vi "Resolve ByteCount Wait.vi"(8 "error in (no error)":errorcluster, 11 "Settings in":T1 {"Channel Refnum" format="%.0x"; "Linked Channels"."Channel Refnum" format="%.0x"}) -> (0 "error out":errorcluster, 1 "Byte Count":i32, 2 "Channel Path":string, 3 "Settings out":T1 {"Channel Refnum" format="%.0x"; "Linked Channels"."Channel Refnum" format="%.0x"})   [LabVIEW 2020, in "Instrument Addon Scripting API.lvlib"]
uses:
  Instrument Addon Scripting API.lvlib
  TypeDefs/ByteCount Response Settings.ctl
  TypeDefs/Linked Channel.ctl
  <vilib>/NI VeriStand/Custom Device API/Custom Device Item Ref.ctl
  NationalInstruments.VeriStand.SystemStorage
  Shared Directory/Instrument Addon Shared.lvlib
  <vilib>/NI VeriStand/Custom Device API/Custom Device API.lvlib
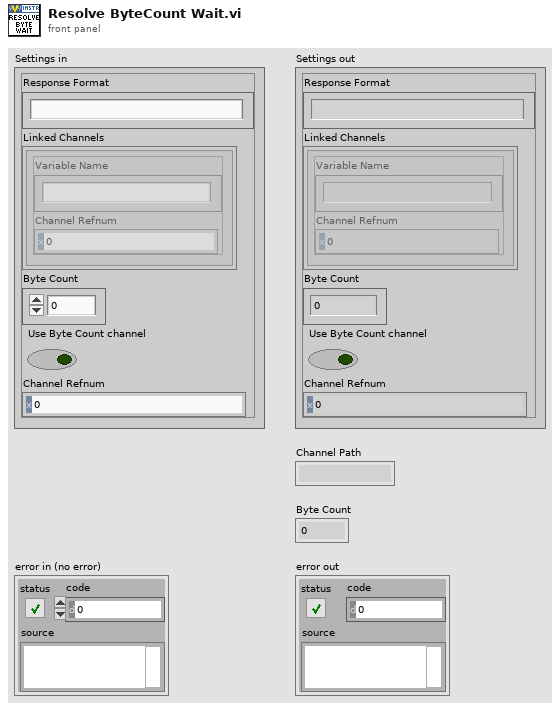
[diagram p1: front panel]
types:
  T1 = typedef "Instrument Addon Scripting API.lvlib/ByteCount Response Settings.ctl" = cluster{"Response Format":string, "Linked Channels":T2[], "Byte Count":i32, "Use Byte Count channel":bool, "Channel Refnum":T3}
  T2 = typedef "Instrument Addon Scripting API.lvlib/Linked Channel.ctl" = cluster{"Variable Name":string, "Channel Refnum":T3}
  T3 = typedef "Custom Device API.lvlib/Custom Device Item Ref.ctl" = u64
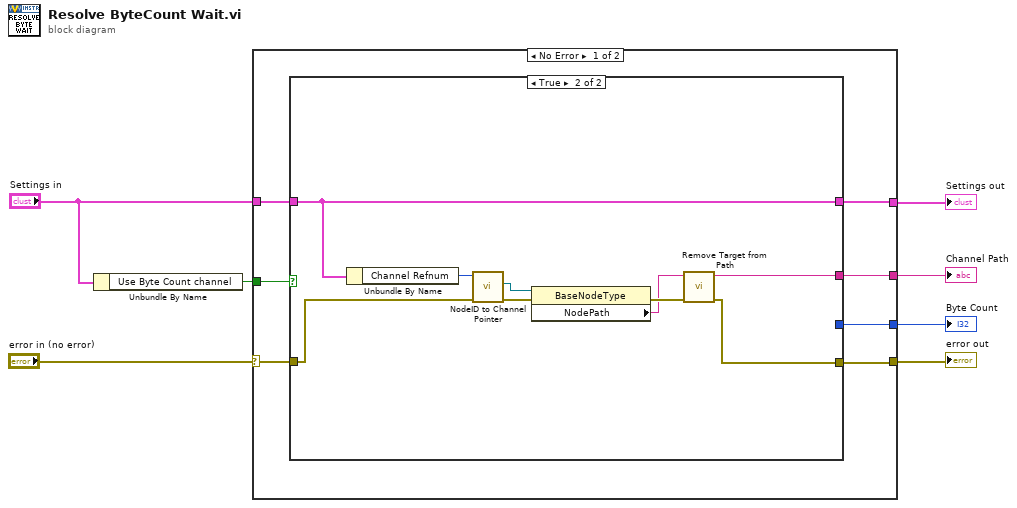
[diagram p0: block diagram]
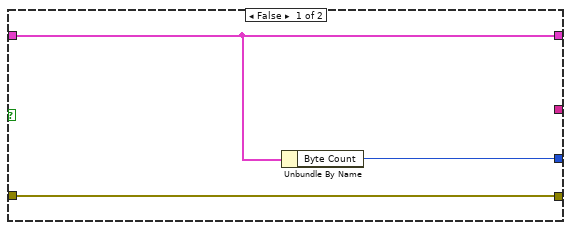
[diagram p2: hidden frame]
diagram:
  n1 = Unbundle By Name("Settings in") -> ("Use Byte Count channel"=w3:bool)
  n2 = case shown="No Error" "error in (no error)" {
    selector: "error in (no error)" -> [w12 w27]
    tunnel: "Settings in" -> [w13 w28]
    tunnel: w3 -> [w14 _]
    tunnel: [w11 w27] -> w7
    tunnel: [w10 w28] -> w6
    tunnel: [w9 _] -> w4
    tunnel: [w8 _] -> w5
    frame No Error {
      n3 = case shown="True" w14 {
        tunnel: w13 -> [w17 w26]
        tunnel: w12 -> [w15 w21]
        tunnel: [w15 w25] -> w11
        tunnel: [w17 w26] -> w10
        tunnel: [_ w24] -> w9
        tunnel: [w16 _] -> w8
        frame False {
          n4 = Unbundle By Name(w17) -> ("Byte Count"=w16:i32)
        }
        frame True {
          n5 = Unbundle By Name(w26) -> ("Channel Refnum"=w20:T3)
          n6 = call "NodeID to Channel Pointer.vi"("error in (no error)"=w21, "nodeID in"=w20) -> ("error out"=w19:errorcluster, "BaseNodeType out"=w18:refnum<k24>)  [unwired: 7 in, 1 out]
          n7 = property class="BaseNodeType"(reference=w18, error in=w19) -> (error out=w23:errorcluster, "NodePath"=w22:string)  [unwired: 1 out]
          n8 = call "Remove Target from Path.vi"("error in (no error)"=w23, "NodePath"=w22) -> ("error out"=w25:errorcluster, "PathArrayToString"=w24:string)  [unwired: 8 in]
        }
      }
    }
    frame Error {
    }
  }
  "error out" <- w7
  "Settings out" <- w6
  "Byte Count" <- w5
  "Channel Path" <- w4
